vi "model-witherrorSD.vi"(1 "Real delay time, ps":dbl) -> (0 "Array":dbl[](array[numeric]))   [LabVIEW 2015]
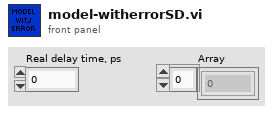
[diagram p1: front panel]
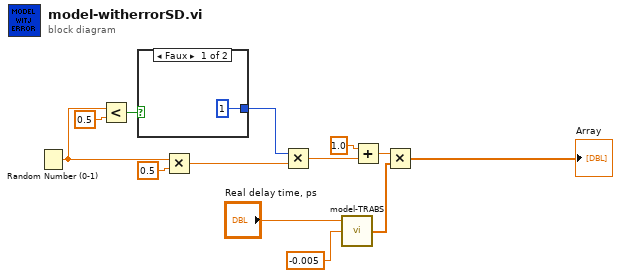
[diagram p0: block diagram]
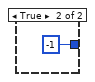
[diagram p2: hidden frame]
diagram:
  n1 = Random Number (0-1)() -> (number: 0 to 1=w1:dbl)
  n2 = Less?(x=w1, y=0.5) -> (x < y?=w8:bool)
  n3 = case shown="Faux" w8 {
    tunnel: [1 -1] -> w10
    frame False {
    }
    frame True {
    }
  }
  n4 = Multiply(x=w1, y=0.5) -> (x*y=w11:dbl)
  n5 = Multiply(x=w10, y=w11) -> (x*y=w12:dbl)
  n6 = call "model-TRABS.vi"("BG"=-0.005, "Real delay time, ps"="Real delay time, ps") -> ("signal out"=w4:dbl[])  [unwired: 1 in]
  n7 = Add(x=1.0, y=w12) -> (x+y=w13:dbl)
  n8 = Multiply(x=w13, y=w4) -> (x*y=→"Array":dbl[])
